vi "oa_Calculate Vector for Given Orders (1 Channel).vi"(0 "resampled signal":cluster{"r0":dbl, "dr":dbl, "Y":dbl[]}={"r0"=0.0, "dr"=1.0, "Y"=[]} {"r0" format="%.2p"; "dr" format="%.2p"; "Y" format="%.2f"}, 1 "reset? (True)":bool=TRUE, 5 "orders to compensate":dbl[](array[numeric])=[1.0] format="%.2f", 7 "slow roll vectors":cdb[](array[numeric]) format="%.2f", 9 "interpolated pulse positions":dbl[](array[numeric]) format="%.2f", 11 "error out in":errorcluster) -> (3 "reset out":bool=TRUE, 6 "orders out":dbl[](array[numeric]) min=0.0 max=127.0 format="%.2f", 8 "slow roll vectors out":cdb[](array[numeric]) format="%.2f", 15 "error out":errorcluster)   [LabVIEW 2017, in "SoundVib_RefDataProcess.lvlib"]
uses:
  <vilib>/addons/Sound and Vibration/Order Analysis/Referece Data Processing/SoundVib_RefDataProcess.lvlib
  <vilib>/addons/Sound and Vibration/Order Analysis/Resample Order Tracking/OAT Order Magnitude and Phase (Even Angle Signal, 1 Channel).vi
  <vilib>/addons/Sound and Vibration/Order Analysis/Resample Order Tracking/SoundVib_OrderTracking.lvlib
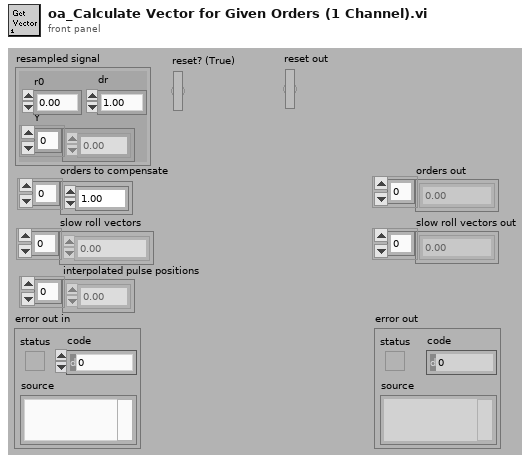
[diagram p1: front panel]
types:
  T1 = cluster{"dB on? (T)":bool, "unwrap phase? (T)":bool, "unit in degree? (T)":bool}
  T2 = cluster{"interpolated pulse positions":dbl[], dbl}
  T3 = typedef "svc_Resampled Channel Info.ctl" = cluster{"channel name":string, "description":string, " channel info":T4}
  T4 = typedef "svc_Channel Info.ctl" = cluster{"sensor sensitivity":dbl, "engineering units":T5, "dB reference":dbl, "custom label":string, "weighting filter":T6, "pregain":dbl}
  T5 = typedef "svc_Engineering Units Text Ring.ctl" = u16
  T6 = typedef "svc_Weighting Filter Text Ring.ctl" = u16
  T7 = cluster{"time/rev/rpm":dbl[], "magnitude":dbl[]}[]
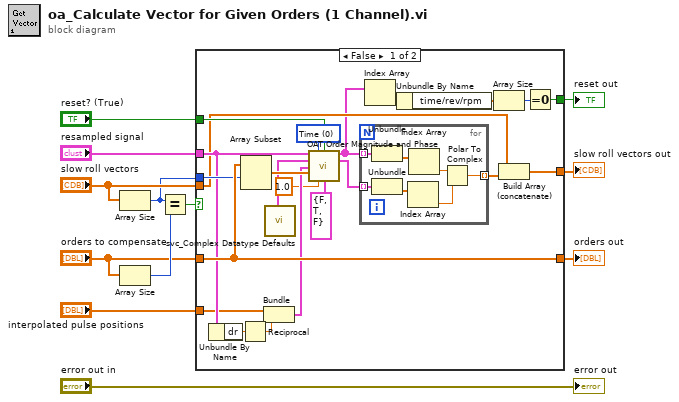
[diagram p0: block diagram]
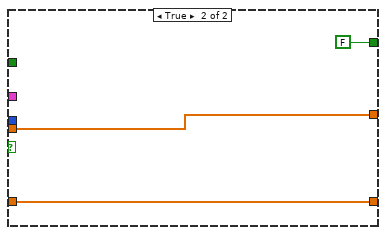
[diagram p2: hidden frame]
diagram:
  n1 = Array Size(array="slow roll vectors") -> (size(s)=w5:i32)
  n2 = Array Size(array="orders to compensate") -> (size(s)=w12:i32)
  n3 = Equal?(x=w5, y=w12) -> (x = y?=w11:bool)
  n4 = case shown="False" w11 {
    tunnel: "slow roll vectors" -> [w22 w44]
    tunnel: [w21 w44] -> w9
    tunnel: "orders to compensate" -> [w34 w43]
    tunnel: [w34 w43] -> w7
    tunnel: w5 -> [w33 _]
    tunnel: "resampled signal" -> [w29 _]
    tunnel: "reset? (True)" -> [w32 _]
    tunnel: "interpolated pulse positions" -> [w26 _]
    tunnel: [w13 FALSE] -> w1
    frame False {
      w31 = u16 0 items=["Time", "Revolution", "RPM"] ("X axis selection")
      n5 = Unbundle By Name(w29) -> ("dr"=w28:dbl)
      n6 = Reciprocal(x=w28) -> (1/x=w25:dbl)
      n7 = Array Subset(array=w34, index=w33) -> (w30:dbl[])  [unwired: 1 in]
      n8 = Bundle("interpolated pulse positions"=w26, w25) -> (w27:T2)  [unwired: 1 in]
      n9 = call <vilib>:"svc_Complex Datatype Defaults.vi"() -> ("resampled channel info"=w18:T3)  [unwired: 11 in, 8 out]
      n10 = call-poly <vilib>:"OAT Order Magnitude and Phase.vi"("even-angle signal"=w29, "x-axis selection"=w31, "reset? (F)"=w32, "even-angle channel info"=w18, "even-angle position info"=w27, "orders to compute (1.0)"=w30, "bandwidth [order]"=1.0, "view"=T1 {"dB on? (T)"=FALSE, "unwrap phase? (T)"=TRUE, "unit in degree? (T)"=FALSE}) -> ("magnitudes [RMS]"=w17:T7, "phases [phase lag]"=w24:cluster{"time/rev/rpm":dbl[], "phase":dbl[]}[])  [unwired: 2 in, 4 out]
      n11 = for {
        tunnel: w17 -> [w41] mode=indexing
        tunnel: w24 -> [w40] mode=indexing
        tunnel: [w39] -> w23 mode=indexing
        n12 = Unbundle(w41) -> ("magnitude"=w38:dbl[])  [unwired: 1 out]
        n13 = Unbundle(w40) -> ("phase"=w36:dbl[])  [unwired: 1 out]
        n14 = Index Array(array=w36) -> (element=w35:dbl)  [unwired: 1 in]
        n15 = Index Array(array=w38) -> (element=w37:dbl)  [unwired: 1 in]
        n16 = Polar To Complex(1:w35, 2:w37) -> (0:w39:cdb)
      }
      n17 = Index Array(array=w17) -> (element=w16:cluster{"time/rev/rpm":dbl[], "magnitude":dbl[]})  [unwired: 1 in]
      n18 = Unbundle By Name(w16) -> ("time/rev/rpm"=w15:dbl[])
      n19 = Array Size(array=w15) -> (size(s)=w14:i32)
      n20 = Build Array (concatenate)(w22, w23) -> (w21:cdb[])
      n21 = Equal To 0?(x=w14) -> (x = 0?=w13:bool)
    }
    frame True {
    }
  }
  "slow roll vectors out" <- w9
  "orders out" <- w7
  "reset out" <- w1
  "error out" <- "error out in"
